vi "Get Follow Wall Target Position.vi"(6 "Forward Distance":dbl=250.0, 8 "Wall left?":bool=TRUE, 9 "Target Distance":dbl=120.0) -> (2 "Target Y (Relative)":dbl=239.35954790726353, 3 "Target X (Relative)":dbl=-109.16575240316062)   [LabVIEW 2017]
uses:
  Globals/Pose.vi
panel:
  out "Wall error":dbl=81.91553376568908
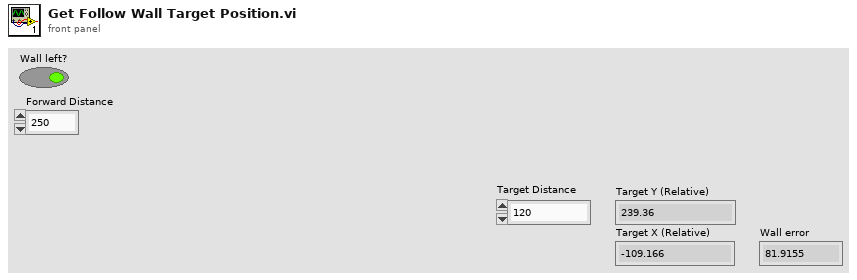
[diagram p1: front panel]
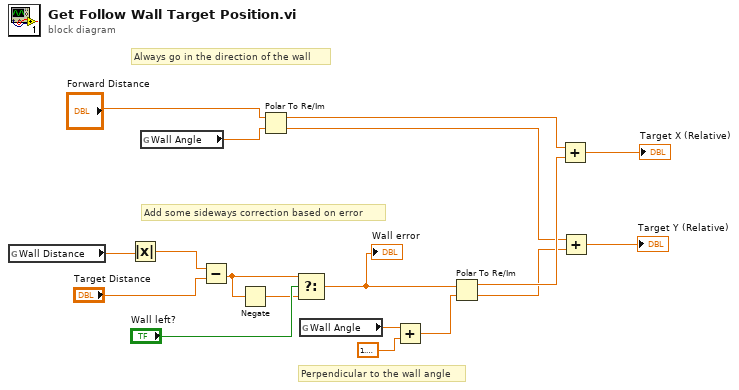
[diagram p0: block diagram]
diagram:
  # "Perpendicular to the wall angle"
  # "Add some sideways correction based on error"
  # "Always go in the direction of the wall"
  n1 = global read "Pose.vi" "Wall Distance"() -> (w3:dbl)
  n2 = Absolute Value(x=w3) -> (abs(x)=w2:dbl)
  n3 = global read "Pose.vi" "Wall Angle"() -> (w18:dbl)
  n4 = Subtract(x=w2, y="Target Distance") -> (x-y=w16:dbl)
  n5 = Negate(x=w16) -> (-x=w15:dbl)
  n6 = Polar To Re/Im(2:w18, 3:"Forward Distance") -> (0:w8:dbl, 1:w10:dbl)
  n7 = Select(t=w16, s="Wall left?", f=w15) -> (s? t:f=w12:dbl)
  "Wall error" <- w12
  n8 = global read "Pose.vi" "Wall Angle"() -> (w14:dbl)
  n9 = Add(x=w14, y=1.5707963267948966) -> (x+y=w11:dbl)
  n10 = Polar To Re/Im(2:w11, 3:w12) -> (0:w7:dbl, 1:w9:dbl)
  n11 = Add(x=w10, y=w9) -> (x+y=→"Target X (Relative)":dbl)
  n12 = Add(x=w8, y=w7) -> (x+y=→"Target Y (Relative)":dbl)
